vi "Pose3d_New_Pose2d.vi"(11 "in POSE2D":T1={"TRANSLATION"={"X"=0.0, "Y"=0.0}, "ROTATION"={"VALUE"=0.0, "COS"=1.0, "SIN"=0.0}} {"ROTATION"."SIN" format="%13.4f"; "ROTATION"."COS" format="%13.4f"; "ROTATION"."VALUE" format="%13.4f"; "TRANSLATION"."Y" format="%14.3f"; "TRANSLATION"."X" format="%14.3f"}) -> (3 "out Pose3d":T4={"Translation3d"={"X"=0.0, "Y"=0.0, "Z"=0.0}, "Rotation3d"={"Q_quaternion"={"R"=1.0, "V"=[0.0, 0.0, 0.0]}}} {"Translation3d"."Z" format="%14.3f"; "Translation3d"."Y" format="%14.3f"; "Translation3d"."X" format="%14.3f"})   [LabVIEW 2019, in "Trajectory_Library.lvlib"]
doc: "Constructs a 3D pose from a 2D pose in the X-Y plane\n\nParameters:\n - in Pose2 -- Pose 2d in the X-Y plane to convert to Pose 3D.\n\nReturns:\n - OUT POSE3D - Output POSE3D"
uses:
  Trajectory_Library.lvlib
  TypeDef/QUATERNION.ctl
  TypeDef/ROTATION3D.ctl
  TypeDef/TRANSLATION3D.ctl
  TypeDef/POSE3D.ctl
  TypeDef/TRANSLATION2D.ctl
  TypeDef/ROTATION2D.ctl
  TypeDef/POSE2D.ctl
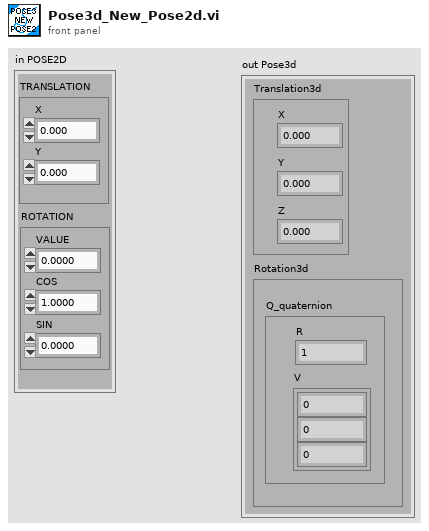
[diagram p1: front panel]
types:
  T1 = typedef "Trajectory_Library.lvlib/POSE2D.ctl" = cluster{"TRANSLATION":T2, "ROTATION":T3}
  T2 = typedef "Trajectory_Library.lvlib/TRANSLATION2D.ctl" = cluster{"X":dbl, "Y":dbl}
  T3 = typedef "Trajectory_Library.lvlib/ROTATION2D.ctl" = cluster{"VALUE":dbl, "COS":dbl, "SIN":dbl}
  T4 = typedef "Trajectory_Library.lvlib/POSE3D.ctl" = cluster{"Translation3d":T5, "Rotation3d":T6}
  T5 = typedef "Trajectory_Library.lvlib/TRANSLATION3D.ctl" = cluster{"X":dbl, "Y":dbl, "Z":dbl}
  T6 = typedef "Trajectory_Library.lvlib/ROTATION3D.ctl" = cluster{"Q_quaternion":T7}
  T7 = typedef "Trajectory_Library.lvlib/QUATERNION.ctl" = cluster{"R":dbl, "V":dbl[]}
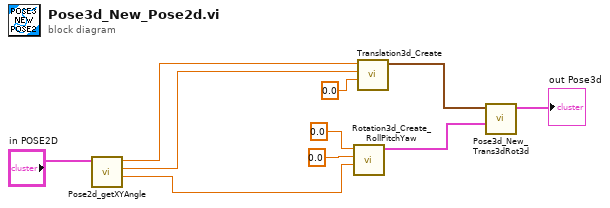
[diagram p0: block diagram]
diagram:
  n1 = call "Pose2d_getXYAngle.vi"("in POSE"="in POSE2D") -> ("Angle"=w1:dbl, "Y"=w2:dbl, "X"=w3:dbl)  [unwired: 8 in]
  n2 = call "Rotation3d_Create_RollPitchYaw.vi"("Yaw"=w1, "Pitch"=0.0, "Roll"=0.0) -> ("Rotation3d"=w8:T6)  [unwired: 8 in]
  n3 = call "Translation3d_Create.vi"("Z"=0.0, "Y"=w2, "X"=w3) -> ("TRANSLATION3D"=w9:T5)  [unwired: 8 in]
  n4 = call "Pose3d_New_Trans3dRot3d.vi"("Rotation3d"=w8, "Translation3d"=w9) -> ("outPose3d"=→"out Pose3d":T4)  [unwired: 9 in]
